vi "Format build_all.bat.vi"(7 "template folder":path, 8 "error in (no error)":errorcluster, 11 "build.bat paths":path[](array[path])) -> (0 "error out":errorcluster, 2 "resulting string":string, 3 "build_all.bat path":path)   [LabVIEW 2019, in "Build.lvlib"]
uses:
  Build/Build.lvlib
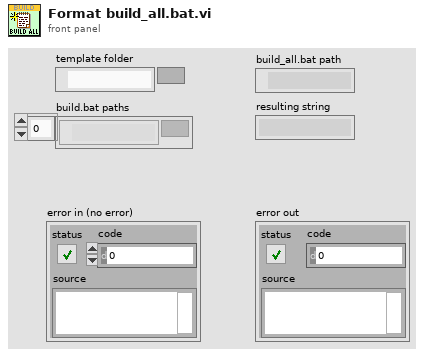
[diagram p1: front panel]
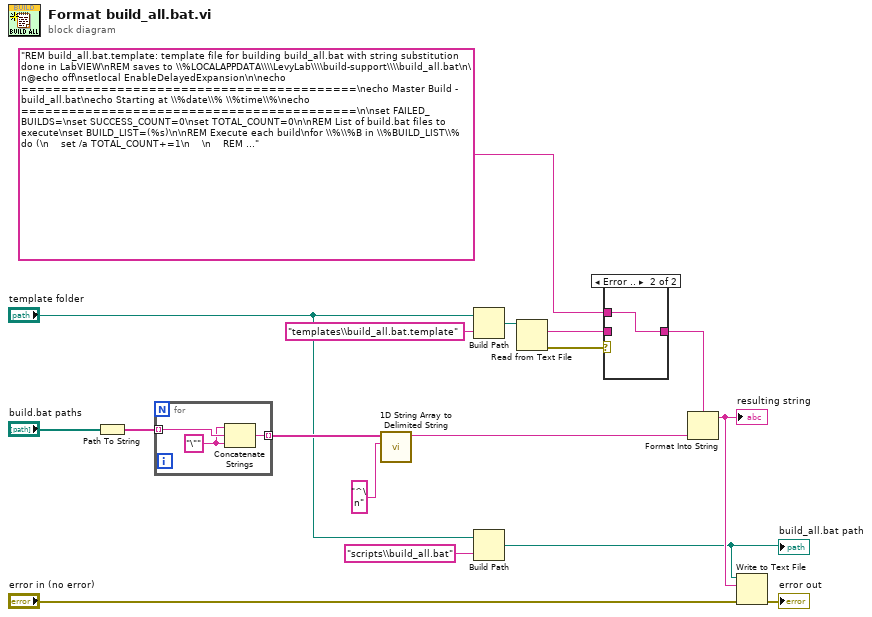
[diagram p0: block diagram]
diagram:
  n1 = Path To String(path="build.bat paths") -> (string=w9:string[])
  n2 = for {
    tunnel: w9 -> [w20] mode=indexing
    tunnel: [w19] -> w10 mode=indexing
    w18 = "\"" ("string")
    n3 = Concatenate Strings(w18, w20, w18) -> (w19:string)
  }
  n4 = call <vilib>:"1D String Array to Delimited String.vi"("delimiter"="^\n", "string array"=w10) -> ("delimited string"=w7:string)  [unwired: 9 in]
  n5 = Build Path(base path="template folder", name or relative path="templates\\build_all.bat.template") -> (appended path=w17:path)
  n6 = Build Path(base path="template folder", name or relative path="scripts\\build_all.bat") -> (appended path=w14:path)
  "build_all.bat path" <- w14
  n7 = Read from Text File(file (use dialog)=w17) -> (text=w3:string, error out=w5:errorcluster)  [unwired: 3 in, 2 out]
  n8 = case shown="Error .." w5 {
    tunnel: [w21 w22] -> w4
    tunnel: w3 -> [w21 _]
    tunnel: "REM build_all.bat.template: template file for building build_all.bat with string substitution done in LabVIEW\nREM saves to \\%LOCALAPPDATA\\\\LevyLab\\\\build-support\\\\build_all.bat\n\n@echo off\nsetlocal EnableDelayedExpansion\n\necho ==========================================\necho Master Build - build_all.bat\necho Starting at \\%date\\% \\%time\\%\necho ==========================================\n\nset FAILED_BUILDS=\nset SUCCESS_COUNT=0\nset TOTAL_COUNT=0\n\nREM List of build.bat files to execute\nset BUILD_LIST=(%s)\n\nREM Execute each build\nfor \\%\\%B in \\%BUILD_LIST\\% do (\n    set /a TOTAL_COUNT+=1\n    \n    REM Extract repo name from path (second-to-last folder)\n    for \\%\\%P in (\"\\%\\%~dpB..\") do set REPO_NAME=\\%\\%~nxP\n    \n    echo.\n    echo ==========================================\n    echo [!TOTAL_COUNT!] Building !REPO_NAME!\n    echo ==========================================\n    \n    REM Change to the build.bat directory and execute\n    cd /d \"\\%\\%~dpB\"\n    call \"\\%\\%~nxB\"\n    \n    if !ERRORLEVEL! neq 0 (\n        echo ERROR: !REPO_NAME! failed\n        set FAILED_BUILDS=!FAILED_BUILDS! !REPO_NAME!\n    ) else (\n        echo SUCCESS: !REPO_NAME!\n        set /a SUCCESS_COUNT+=1\n    )\n)\n\nREM Summary\necho.\necho ==========================================\necho Build Summary\necho ==========================================\necho Total: \\%TOTAL_COUNT\\%\necho Success: \\%SUCCESS_COUNT\\%\n\nif \"\\%FAILED_BUILDS\\%\"==\"\" (\n    echo All builds completed successfully!\n    exit /b 0\n) else (\n    echo Failed builds:\\%FAILED_BUILDS\\%\n    exit /b 1\n)" -> [_ w22]
    frame No Error {
    }
    frame Error {
    }
  }
  n9 = Format Into String(format string=w4, w7) -> (resulting string=w15:string)  [unwired: 2 in, 1 out]
  "resulting string" <- w15
  n10 = Write to Text File(file (use dialog)=w14, text=w15, error in="error in (no error)") -> (error out=→"error out":errorcluster)  [unwired: 1 in, 2 out]
